vi "PostInstall.vi"(10 "Variant":variant) -> (0 "error out":errorcluster)   [LabVIEW 2016]
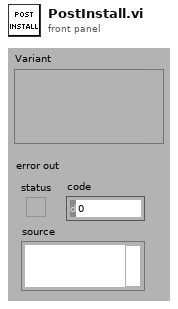
[diagram p1: front panel]
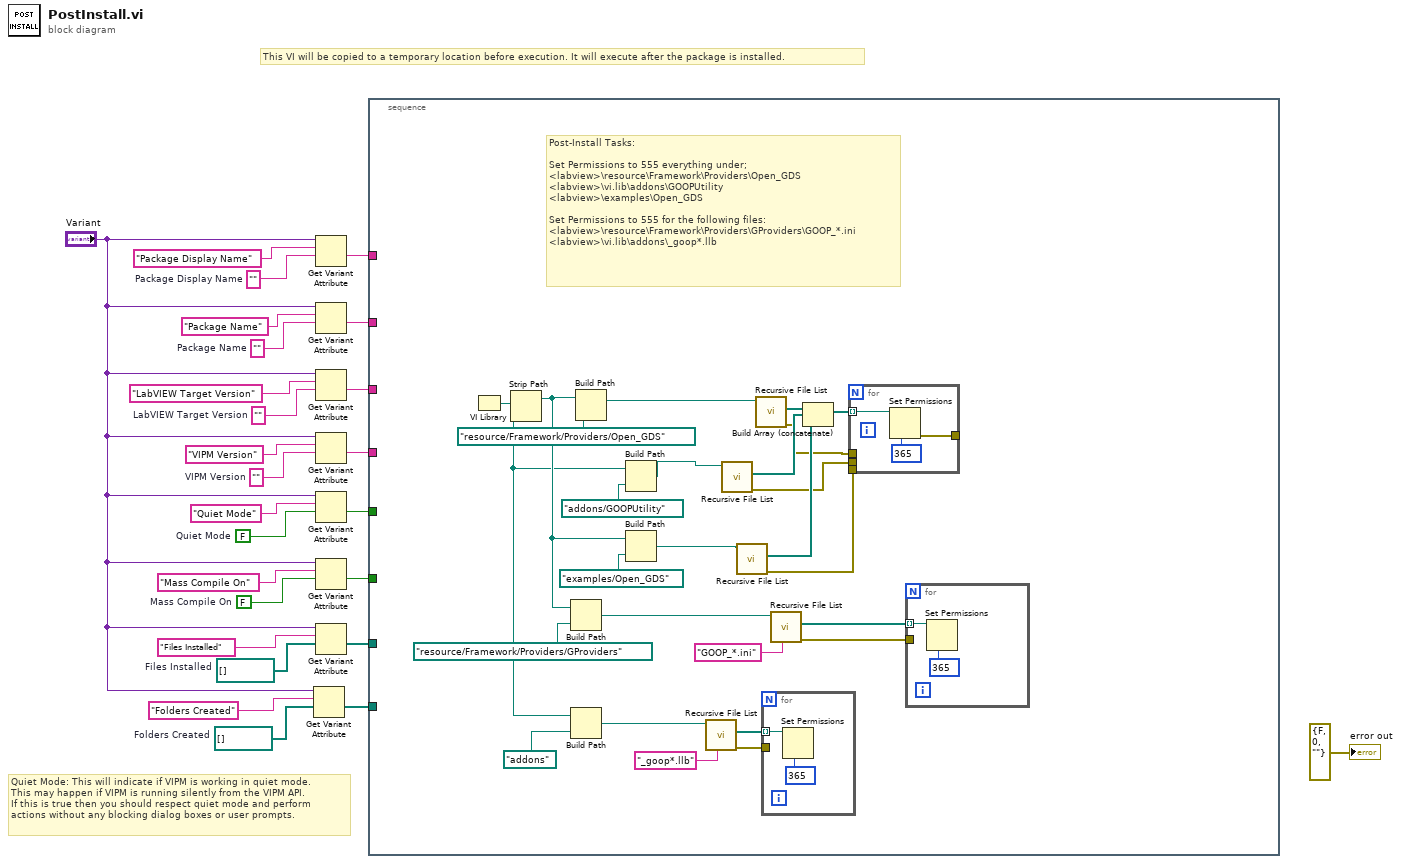
[diagram p0: block diagram]
diagram:
  w1 = path[] []  # Folders Created
  w2 = path[] []  # Files Installed
  w8 = FALSE  # Mass Compile On
  w9 = ""  # Package Display Name
  w16 = FALSE  # Quiet Mode
  w19 = ""  # VIPM Version
  w21 = ""  # LabVIEW Target Version
  w23 = ""  # Package Name
  # "Quiet Mode: This will indicate if VIPM is working in quiet mode.\nThis may happen if VIPM is running silently from the VIPM API.\nIf this is true then you should respect quiet mode and perform\nactions without any blocking dialog boxes or user prompts."
  # "This VI will be copied to a temporary location before execution. It will execute after the package is installed."
  n1 = Get Variant Attribute(Variant="Variant", name="Folders Created", default value (empty Variant)=w1) -> (value=w6:path[])  [unwired: 1 in, 3 out]
  n2 = Get Variant Attribute(Variant="Variant", name="Package Display Name", default value (empty Variant)=w9) -> (value=w15:string)  [unwired: 1 in, 3 out]
  n3 = Get Variant Attribute(Variant="Variant", name="Package Name", default value (empty Variant)=w23) -> (value=w14:string)  [unwired: 1 in, 3 out]
  n4 = Get Variant Attribute(Variant="Variant", name="LabVIEW Target Version", default value (empty Variant)=w21) -> (value=w13:string)  [unwired: 1 in, 3 out]
  n5 = Get Variant Attribute(Variant="Variant", name="VIPM Version", default value (empty Variant)=w19) -> (value=w12:string)  [unwired: 1 in, 3 out]
  n6 = Get Variant Attribute(Variant="Variant", name="Quiet Mode", default value (empty Variant)=w16) -> (value=w11:bool)  [unwired: 1 in, 3 out]
  n7 = Get Variant Attribute(Variant="Variant", name="Mass Compile On", default value (empty Variant)=w8) -> (value=w10:bool)  [unwired: 1 in, 3 out]
  n8 = Get Variant Attribute(Variant="Variant", name="Files Installed", default value (empty Variant)=w2) -> (value=w5:path[])  [unwired: 1 in, 3 out]
  n9 = stacked-sequence {
    tunnel: w15 -> [_]
    tunnel: w14 -> [_]
    tunnel: w13 -> [_]
    tunnel: w12 -> [_]
    tunnel: w11 -> [_]
    tunnel: w10 -> [_]
    tunnel: w5 -> [_]
    tunnel: w6 -> [_]
    frame #0 {
      # "Post-Install Tasks:\n\nSet Permissions to 555 everything under;\n<labview>\\resource\\Framework\\Providers\\Open_GDS\n<labview>\\vi.lib\\addons\\GOOPUtility\n<labview>\\examples\\Open_GDS\n\nSet Permissions to 555 for the following files:\n<labview>\\resource\\Framework\\Providers\\GProviders\\GOOP_*.ini\n<labview>\\vi.lib\\addons\\_goop*.llb"
      n10 = VI Library() -> (path=w34:path)
      n11 = Strip Path(path=w34) -> (stripped path=w43:path)  [unwired: 1 out]
      n12 = Build Path(base path=w43, name or relative path=path "resource/Framework/Providers/GProviders" ("path")) -> (appended path=w39:path)
      n13 = Build Path(base path=w34, name or relative path=path "addons" ("path")) -> (appended path=w35:path)
      n14 = Build Path(base path=w43, name or relative path=path "resource/Framework/Providers/Open_GDS" ("path")) -> (appended path=w48:path)
      n15 = Build Path(base path=w34, name or relative path=path "addons/GOOPUtility" ("path")) -> (appended path=w42:path)
      n16 = Build Path(base path=w43, name or relative path=path "examples/Open_GDS" ("path")) -> (appended path=w41:path)
      n17 = call <vilib>:"Recursive File List.vi"("pattern"="_goop*.llb", "Folder Path"=w35) -> ("error out"=w27:errorcluster, "All Files in Dir"=w32:path[])  [unwired: 5 in, 3 out]
      n18 = call <vilib>:"Recursive File List.vi"("Folder Path"=w42) -> ("error out"=w30:errorcluster, "All Files in Dir"=w45:path[])  [unwired: 6 in, 3 out]
      n19 = call <vilib>:"Recursive File List.vi"("Folder Path"=w41) -> ("error out"=w29:errorcluster, "All Files in Dir"=w40:path[])  [unwired: 6 in, 3 out]
      n20 = call <vilib>:"Recursive File List.vi"("Folder Path"=w48) -> ("error out"=w31:errorcluster, "All Files in Dir"=w50:path[])  [unwired: 6 in, 3 out]
      n21 = for {
        tunnel: w32 -> [w52] mode=indexing
        tunnel: w27 -> [_]
        n22 = Set Permissions(7:i16 365 ("permissions"), 11:w52) -> ()  [unwired: 3 in, 2 out]
      }
      n23 = call <vilib>:"Recursive File List.vi"("pattern"="GOOP_*.ini", "Folder Path"=w39) -> ("error out"=w28:errorcluster, "All Files in Dir"=w37:path[])  [unwired: 5 in, 3 out]
      n24 = Build Array (concatenate)(w50, w45, w40) -> (w49:path[])
      n25 = for {
        tunnel: w49 -> [w56] mode=indexing
        tunnel: [w54] -> _
        tunnel: w31 -> [_]
        tunnel: w30 -> [_]
        tunnel: w29 -> [_]
        n26 = Set Permissions(7:i16 365 ("permissions"), 11:w56) -> (0:w54:errorcluster)  [unwired: 3 in, 1 out]
      }
      n27 = for {
        tunnel: w37 -> [w57] mode=indexing
        tunnel: w28 -> [_]
        n28 = Set Permissions(7:i16 365 ("permissions"), 11:w57) -> ()  [unwired: 3 in, 2 out]
      }
    }
  }
  "error out" <- errorcluster {"status"=FALSE, "code"=0, "source"=""} ("error out")
